vi "Four loops-one value from inner loop-HuYang.vi"(0 "File or Folder Path":path=path "P:/expt/PPMS data/SA03074H.20180120/14-rf1-rf2-9T", 5 "offset for each\n SG1 loop":i32, 7 "length X":i32=126, 9 "index":T1={"A"=10, "B"=1, "C"=2, "D"=0, "E"=10, "N1"=0, "N2"=0, "N3"=0, "N4"=0}, 11 "stop":bool, 12 "file contains 2D data?":bool) -> (4 "A vs B":cluster{i32[], dbl[]}[](graph), 6 "C vs D":cluster{dbl[], dbl[]}[](graph), 8 "E":dbl[][](graph), 10 "N":cluster{"N1":dbl, "N2":dbl, "N3":dbl, "N4":dbl}={"N1"=3599514757.669291, "N2"=3599514757.669291, "N3"=3599514757.669291, "N4"=3599514757.669291} {"N4" format="%#_6p"; "N3" format="%#_6p"; "N2" format="%#_6p"; "N1" format="%#_6p"}, 14 "Comments":string="IGOR\nX// Date: 1/22/2018 8:13 PM\nX// //Changed Voltage Femto from 20 dB to 80 dB (lock in channel 2)\nX// \nX// Stability diagram sweep\nX// \nX// Bias sweep: 0mV to 5mV, 2.5mV\nX// RF level sweep: - 4dBm, 2dBm\nX// DC2: -100 mV to 150mV, 2mV step\nX// DC1: -100 mV to 250mV, 1mV step\nX// \nX// B = 9T\nX// T = 50 mK\nX// Backgate = -0.1V \nX// \nX// I+: 5   0Vac + dc sweep, 13Hz, Sine wave\nX// I-: 28\nX// \nX// V1+/-: 4/27\nX// V2+/-: NA\nX// V3+/V3-: NA\nX// Vsg: 2&3\nX// \nX// 60 Hz prefilter off\nX// TC: 50m\nX// order:2\nX// SR830m sensitivity: 500uV\nX// \nX// I input gain: 1E+6\nX// V input gain:  10000appliedVsg= 0.000000\nX// appliedT= -4.000000appliedVsg= 0.150000\n\n\n\n\n\n\n\n\n\n\n\n\n\n\n\n\n\n\n\n\n\n\n\n\n\n\n\n\n\n\n\n\n\n\n\n\n\n\n\n\n\n\n\n\n\n\n\n\n\n\n\n\n\n\n\n\n\n\n\n\n\n\nX \nX Display/R 'time.SA03074H.000125'\nX AppendToGraph 'Vsg.SA03074H.000125'\nX AppendToGraph 'T.SA03074H.000125'\nX AppendToGraph 'B.SA03074H.000125'\nX AppendToGraph 'X0.SA03074H.000125'\nX AppendToGraph 'Y0.SA03074H.000125'\nX AppendToGraph 'X1.SA03074H.000125'\nX AppendToGraph 'Y1.SA03074H.000125'\nX AppendToGraph 'X2.SA03074H.000125'\nX AppendToGraph 'Y2.SA03074H.000125'\nX AppendToGraph 'X3.SA03074H.000125'\nX AppendToGraph 'Y3.SA03074H.000125'\nX AppendToGraph 'X4.SA03074H.000125'\nX AppendToGraph 'Y4.SA03074H.000125'\nX AppendToGraph 'X5.SA03074H.000125'\nX AppendToGraph 'Y5.SA03074H.000125'\nX AppendToGraph 'X6.SA03074H.000125'\nX AppendToGraph 'Y6.SA03074H.000125'\nX AppendToGraph 'X7.SA03074H.000125'\nX AppendToGraph 'Y7.SA03074H.000125'\nX AppendToGraph 'X8.SA03074H.000125'\nX AppendToGraph 'Y8.SA03074H.000125'\nX AppendToGraph 'X9.SA03074H.000125'\nX AppendToGraph 'Y9.SA03074H.000125'\nX AppendToGraph 'Gcalc.SA03074H.000125'\nX AppendToGraph '25.SA03074H.000125'\nX AppendToGraph '26.SA03074H.000125'\nX AppendToGraph '27.SA03074H.000125'\nX AppendToGraph '28.SA03074H.000125'\nX AppendToGraph '29.SA03074H.000125'\nX Label bottom \"x label\"\nX Label left \"y label\"\nX ModifyGraph rgb('time.SA03074H.000125')=(65280,0,0)\nX ModifyGraph rgb('Vsg.SA03074H.000125')=(65280,12288,0)\nX ModifyGraph rgb('T.SA03074H.000125')=(65280,23040,0)\nX ModifyGraph rgb('B.SA03074H.000125')=(65280,35328,0)\nX ModifyGraph rgb('X0.SA03074H.000125')=(65280,47616,0)\nX ModifyGraph rgb('Y0.SA03074H.000125')=(65280,58368,0)\nX ModifyGraph rgb('X1.SA03074H.000125')=(60416,65280,0)\nX ModifyGraph rgb('Y1.SA03074H.000125')=(48128,65280,0)\nX ModifyGraph rgb('X2.SA03074H.000125')=(37376,65280,0)\nX ModifyGraph rgb('Y2.SA03074H.000125')=(25088,65280,0)\nX ModifyGraph rgb('X3.SA03074H.000125')=(12800,65280,0)\nX ModifyGraph rgb('Y3.SA03074H.000125')=(2048,65280,0)\nX ModifyGraph rgb('X4.SA03074H.000125')=(0,65280,10240)\nX ModifyGraph rgb('Y4.SA03074H.000125')=(0,65280,22528)\nX ModifyGraph rgb('X5.SA03074H.000125')=(0,65280,33280)\nX ModifyGraph rgb('Y5.SA03074H.000125')=(0,65280,45568)\nX ModifyGraph rgb('X6.SA03074H.000125')=(0,65280,57856)\nX ModifyGraph rgb('Y6.SA03074H.000125')=(0,62464,65280)\nX ModifyGraph rgb('X7.SA03074H.000125')=(0,50176,65280)\nX ModifyGraph rgb('Y7.SA03074H.000125')=(0,37888,65280)\nX ModifyGraph rgb('X8.SA03074H.000125')=(0,27136,65280)\nX ModifyGraph rgb('Y8.SA03074H.000125')=(0,14848,65280)\nX ModifyGraph rgb('X9.SA03074H.000125')=(0,2560,65280)\nX ModifyGraph rgb('Y9.SA03074H.000125')=(8192,0,65280)\nX ModifyGraph rgb('Gcalc.SA03074H.000125')=(20480,0,65280)\nX ModifyGraph rgb('25.SA03074H.000125')=(32768,0,65280)\nX ModifyGraph rgb('26.SA03074H.000125')=(43520,0,65280)\nX ModifyGraph rgb('27.SA03074H.000125')=(55808,0,65280)\nX ModifyGraph rgb('28.SA03074H.000125')=(65280,0,62976)\nX ModifyGraph rgb('29.SA03074H.000125')=(65280,0,52224)\nX Legend/C/N=text0/J \"\\\\s('time.SA03074H.000125') time\\r\\\\s('Vsg.SA03074H.000125') Vsg\\r\\\\s('T.SA03074H.000125') T\\r\\\\s('B.SA03074H.000125') B\\r\\\\s('X0.SA03074H.000125') X0\\r\\\\s('Y0.SA03074H.000125') Y0\\r\\\\s('X1.SA03074H.000125') X1\\r\\\\s('Y1.SA03074H.000125') Y1\\r\\\\s('X2.SA03074H.000125') X2\\r\\\\s('Y2.SA03074H.000125') Y2\\r\\\\s('X3.SA03074H.000125') X3\\r\\\\s('Y3.SA03074H.000125') Y3\\r\\\\s('X4.SA03074H.000125') X4\\r\\\\s('Y4.SA03074H.000125') Y4\\r\\\\s('X5.SA03074H.000125') X5\\r\\\\s('Y5.SA03074H.000125') Y5\\r\\\\s('X6.SA03074H.000125') X6\\r\\\\s('Y6.SA03074H.000125') Y6\\r\\\\s('X7.SA03074H.000125') X7\\r\\\\s('Y7.SA03074H.000125') Y7\\r\\\\s('X8.SA03074H.000125') X8\\r\\\\s('Y8.SA03074H.000125') Y8\\r\\\\s('X9.SA03074H.000125') X9\\r\\\\s('Y9.SA03074H.000125') Y9\\r\\\\s('Gcalc.SA03074H.000125') Gcalc\"\nX ModifyGraph mirror(bottom)=1\nX ModifyGraph width=216\nX ModifyGraph height={Aspect,0.6}\nX ModifyGraph Log(bottom)=0\nX ModifyGraph Log(left)=0\nX \n")   [LabVIEW 2016]
uses:
  <vilib>/Utility/miscctls.llb/LVOffsetAndMultiplierTypeDef.ctl
panel:
  in  "length Y":i32
  in  "Index of inner loop":i32
  in  "D  is time?":bool
  in  "B is time?":bool
  out "time":string[][](table)=[["1/22/2018", "5:40 PM"], ["1/22/2018", "5:41 PM"], ["1/22/2018", "5:42 PM"], ["1/22/2018", "5:43 PM"], ["1/22/2018", "5:44 PM"], ["1/22/2018", "5:46 PM"], ["1/22/2018", "5:47 PM"], ["1/22/2018", "5:48 PM"], ["1/22/2018", "5:49 PM"], ["1/22/2018", "5:51 PM"], ["1/22/2018", "5:52 PM"], ["1/22/2018", "5:53 PM"], ["1/22/2018", "5:54 PM"], ["1/22/2018", "5:55 PM"], ["1/22/2018", "5:57 PM"], ["1/22/2018", "5:58 PM"], ["1/22/2018", "5:59 PM"], ["1/22/2018", "6:00 PM"], ["1/22/2018", "6:02 PM"], ["1/22/2018", "6:03 PM"], ["1/22/2018", "6:04 PM"], ["1/22/2018", "6:05 PM"], ["1/22/2018", "6:07 PM"], ["1/22/2018", "6:08 PM"], ["1/22/2018", "6:09 PM"], ["1/22/2018", "6:10 PM"], ["1/22/2018", "6:11 PM"], ["1/22/2018", "6:13 PM"], ["1/22/2018", "6:14 PM"], ["1/22/2018", "6:15 PM"], ["1/22/2018", "6:16 PM"], ["1/22/2018", "6:18 PM"], ["1/22/2018", "6:19 PM"], ["1/22/2018", "6:20 PM"], ["1/22/2018", "6:21 PM"], ["1/22/2018", "6:23 PM"], ["1/22/2018", "6:24 PM"], ["1/22/2018", "6:25 PM"], ["1/22/2018", "6:26 PM"], ["1/22/2018", "6:27 PM"], ["1/22/2018", "6:29 PM"], ["1/22/2018", "6:30 PM"], ["1/22/2018", "6:31 PM"], ["1/22/2018", "6:32 PM"], ["1/22/2018", "6:34 PM"], ["1/22/2018", "6:35 PM"], ["1/22/2018", "6:36 PM"], ["1/22/2018", "6:37 PM"], ["1/22/2018", "6:39 PM"], ["1/22/2018", "6:40 PM"], ["1/22/2018", "6:41 PM"], ["1/22/2018", "6:42 PM"], ["1/22/2018", "6:43 PM"], ["1/22/2018", "6:45 PM"], ["1/22/2018", "6:46 PM"], ["1/22/2018", "6:47 PM"], ["1/22/2018", "6:48 PM"], ["1/22/2018", "6:50 PM"], ["1/22/2018", "6:51 PM"], ["1/22/2018", "6:52 PM"], ["1/22/2018", "6:53 PM"], ["1/22/2018", "6:55 PM"], ["1/22/2018", "6:56 PM"], ["1/22/2018", "6:57 PM"], ["1/22/2018", "6:58 PM"], ["1/22/2018", "6:59 PM"], ["1/22/2018", "7:01 PM"], ["1/22/2018", "7:02 PM"], ["1/22/2018", "7:03 PM"], ["1/22/2018", "7:04 PM"], ["1/22/2018", "7:06 PM"], ["1/22/2018", "7:07 PM"], ["1/22/2018", "7:08 PM"], ["1/22/2018", "7:09 PM"], ["1/22/2018", "7:11 PM"], ["1/22/2018", "7:12 PM"], ["1/22/2018", "7:13 PM"], ["1/22/2018", "7:14 PM"], ["1/22/2018", "7:15 PM"], ["1/22/2018", "7:17 PM"], ["1/22/2018", "7:18 PM"], ["1/22/2018", "7:19 PM"], ["1/22/2018", "7:20 PM"], ["1/22/2018", "7:22 PM"], ["1/22/2018", "7:23 PM"], ["1/22/2018", "7:24 PM"], ["1/22/2018", "7:25 PM"], ["1/22/2018", "7:27 PM"], ["1/22/2018", "7:28 PM"], ["1/22/2018", "7:29 PM"], ["1/22/2018", "7:30 PM"], ["1/22/2018", "7:32 PM"], ["1/22/2018", "7:33 PM"], ["1/22/2018", "7:34 PM"], ["1/22/2018", "7:35 PM"], ["1/22/2018", "7:36 PM"], ["1/22/2018", "7:38 PM"], ["1/22/2018", "7:39 PM"], ["1/22/2018", "7:40 PM"], ["1/22/2018", "7:41 PM"], ["1/22/2018", "7:43 PM"], ["1/22/2018", "7:44 PM"], ["1/22/2018", "7:45 PM"], ["1/22/2018", "7:46 PM"], ["1/22/2018", "7:48 PM"], ["1/22/2018", "7:49 PM"], ["1/22/2018", "7:50 PM"], ["1/22/2018", "7:51 PM"], ["1/22/2018", "7:52 PM"], ["1/22/2018", "7:54 PM"], ["1/22/2018", "7:55 PM"], ["1/22/2018", "7:56 PM"], ["1/22/2018", "7:57 PM"], ["1/22/2018", "7:59 PM"], ["1/22/2018", "8:00 PM"], ["1/22/2018", "8:01 PM"], ["1/22/2018", "8:02 PM"], ["1/22/2018", "8:04 PM"], ["1/22/2018", "8:05 PM"], ["1/22/2018", "8:06 PM"], ["1/22/2018", "8:07 PM"], ["1/22/2018", "8:08 PM"], ["1/22/2018", "8:10 PM"], ["1/22/2018", "8:11 PM"], ["1/22/2018", "8:12 PM"], ["1/22/2018", "8:13 PM"]]
  in  "Use Folder Index File?":bool
  in  "Generate Folder Index File?":bool
  in  "Ez name":string="Ix (nA)"
  in  "Ey name":string="DC2 (V)"
  in  "Ex name":string="DC1 (V)"
  in  "C y name":string="C y name"
  in  "D x name":string="D x name"
  in  "A y name":string="Ix (nA)"
  in  "B x name":string="DC1 (V)"
  out "Index, Wavenames":string[][](table)=[["0", "'time.SA03074H.000125'\n"], ["1", "'Vsg.SA03074H.000125'\n"], ["2", "'T.SA03074H.000125'\n"], ["3", "'B.SA03074H.000125'\n"], ["4", "'X0.SA03074H.000125'\n"], ["5", "'Y0.SA03074H.000125'\n"], ["6", "'X1.SA03074H.000125'\n"], ["7", "'Y1.SA03074H.000125'\n"], ["8", "'X2.SA03074H.000125'\n"], ["9", "'Y2.SA03074H.000125'\n"], ["10", "'X3.SA03074H.000125'\n"], ["11", "'Y3.SA03074H.000125'\n"], ["12", "'X4.SA03074H.000125'\n"], ["13", "'Y4.SA03074H.000125'\n"], ["14", "'X5.SA03074H.000125'\n"], ["15", "'Y5.SA03074H.000125'\n"], ["16", "'X6.SA03074H.000125'\n"], ["17", "'Y6.SA03074H.000125'\n"], ["18", "'X7.SA03074H.000125'\n"], ["19", "'Y7.SA03074H.000125'\n"], ["20", "'X8.SA03074H.000125'\n"], ["21", "'Y8.SA03074H.000125'\n"], ["22", "'X9.SA03074H.000125'\n"], ["23", "'Y9.SA03074H.000125'\n"], ["24", "'Gcalc.SA03074H.000125'\n"], ["25", "'25.SA03074H.000125'\n"], ["26", "'26.SA03074H.000125'\n"], ["27", "'27.SA03074H.000125'\n"], ["28", "'28.SA03074H.000125'\n"], ["29", "'29.SA03074H.000125'\n"], ["", ""]]
  in  "recolor traces?":bool
  in  "Ex":T2={"Offset"=-0.1, "Multiplier"=0.001}
  in  "Ey":T2={"Offset"=-0.1, "Multiplier"=0.002}
  out "Path":path=path "P:/expt/PPMS data/SA03074H.20180120/14-rf1-rf2-9T/SA03074H.000125.itx"
  out "counter":i32=125
  in  "pattern":string="*.itx"
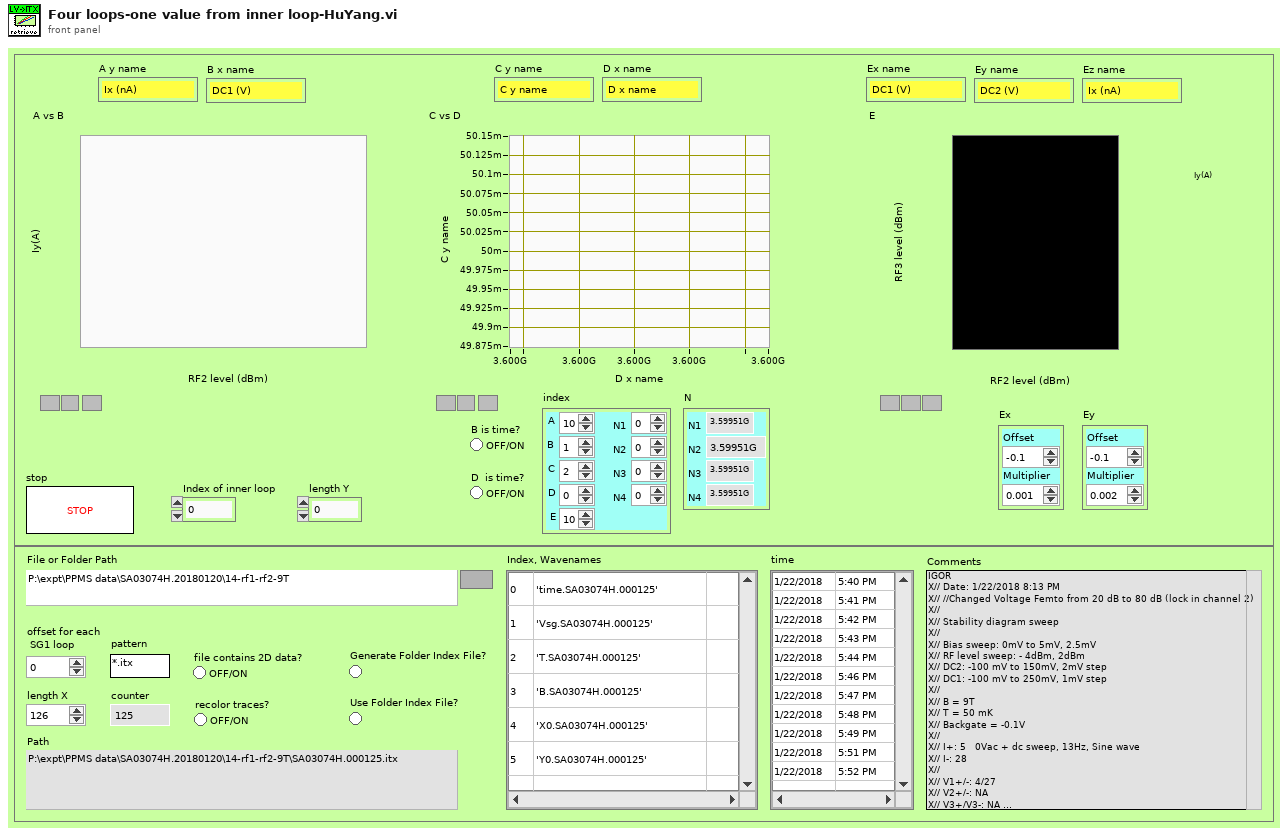
[diagram p1: front panel]
types:
  T1 = cluster{"A":i32, "B":i32, "C":i32, "D":i32, "E":i32, "N1":i32, "N2":i32, "N3":i32, "N4":i32}
  T2 = typedef "LVOffsetAndMultiplierTypeDef.ctl" = cluster{"Offset":dbl, "Multiplier":dbl}
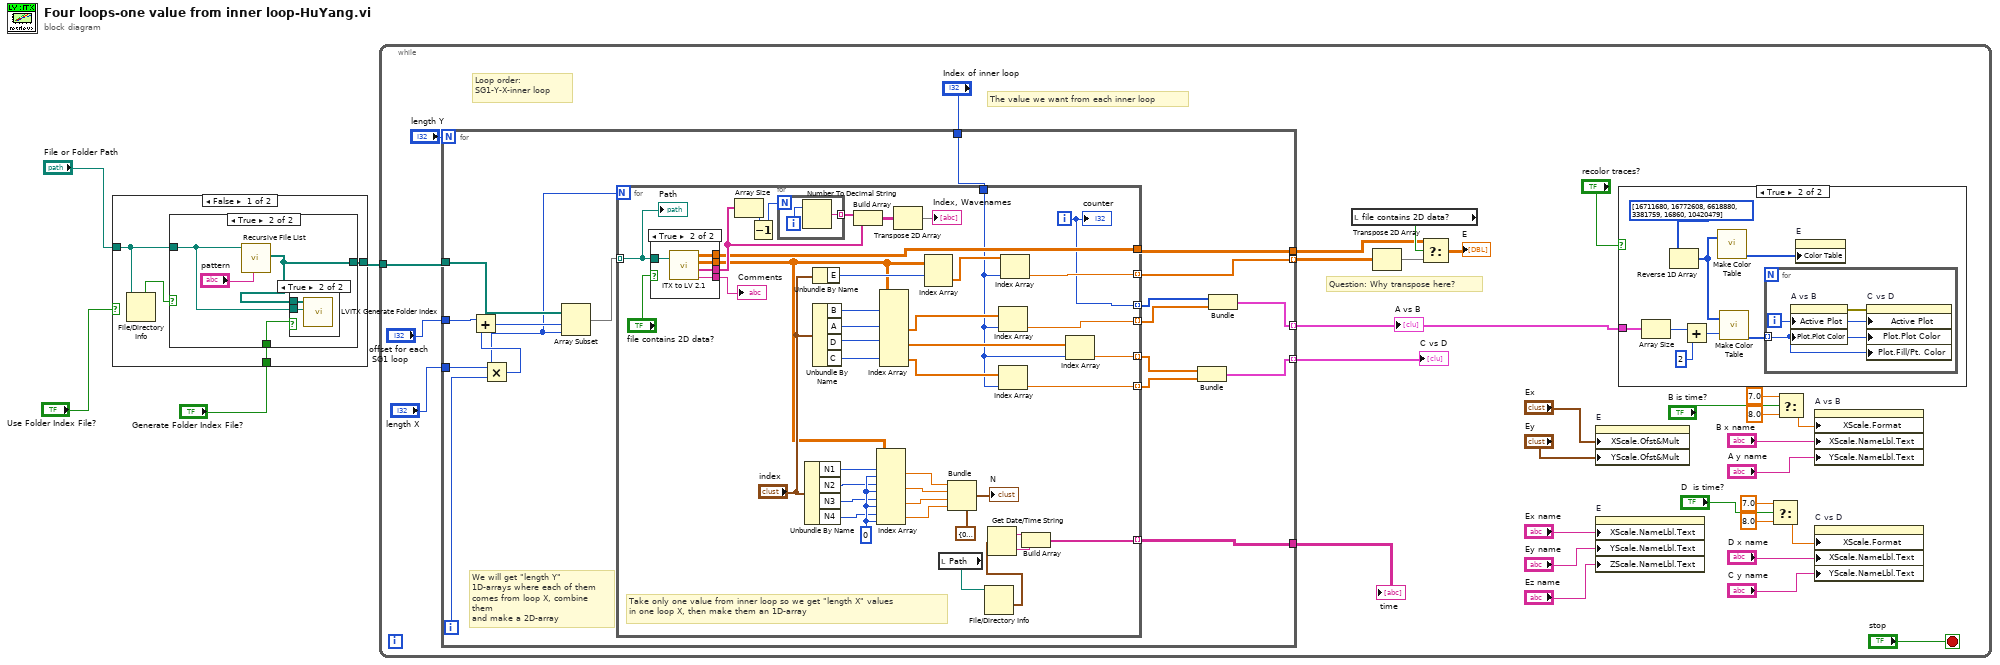
[diagram p0: block diagram]
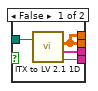
[diagram p2: hidden frame]
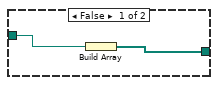
[diagram p4: hidden frame]
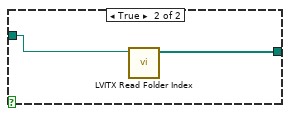
[diagram p6: hidden frame]
diagram:
  n1 = case shown="False" "Use Folder Index File?" {
    tunnel: [w6 w17] -> w2
    tunnel: "File or Folder Path" -> [w8 w18]
    tunnel: "Generate Folder Index File?" -> [w5 _]
    frame False {
      n2 = File/Directory Info(path=w8) -> (directory=w7:bool)  [unwired: 1 in, 6 out]
      n3 = case shown="True" w7 {
        tunnel: [w10 w13] -> w6
        tunnel: w8 -> [w9 w12]
        tunnel: w5 -> [_ w11]
        frame False {
          n4 = Build Array(w9) -> (w10:path[])
        }
        frame True {
          n5 = call <vilib>:"Recursive File List.vi"("pattern"="pattern", "Folder Path"=w12) -> ("All Files in Dir"=w13:path[])  [unwired: 5 in, 4 out]
          n6 = case shown="True" w11 {
            tunnel: w13 -> [_ w16]
            tunnel: w12 -> [_ w15]
            frame False {
            }
            frame True {
              n7 = call <userlib>:"LVITX Generate Folder Index.vi"("File or Folder Path"=w15, "All Files in Dir"=w16) -> ()  [unwired: 10 in]
            }
          }
        }
      }
    }
    frame True {
      n8 = call <userlib>:"LVITX Read Folder Index.vi"("File or Folder Path"=w18) -> ("Array"=w17:path[])  [unwired: 10 in]
    }
  }
  n9 = while {
    tunnel: w2 -> [w22]
    stop <- "stop" stop-if-true
    # "Question: Why transpose here?"
    # "The value we want from each inner loop"
    # "Loop order:\nSG1-Y-X-inner loop"
    n10 = for {
      N: "length Y" -> [_]
      tunnel: [w58] -> w46 mode=indexing
      tunnel: [w67] -> w44
      tunnel: [w57] -> w42 mode=indexing
      tunnel: [w56] -> w41 mode=indexing
      tunnel: [w66] -> w33
      tunnel: w22 -> [w64]
      tunnel: "Index of inner loop" -> [w65]
      tunnel: "offset for each\n SG1 loop" -> [w62]
      tunnel: "length X" -> [w59]
      i -> [w53]
      # "We will get \"length Y\" 1D-arrays where each of them comes from loop X, combine them \nand make a 2D-array"
      n11 = Multiply(x=w59, y=w53) -> (x*y=w63:i32)
      n12 = Add(x=w62, y=w63) -> (x+y=w61:i32)
      n13 = Array Subset(array=w64, index=w61, length=w59) -> (w60:path[])
      n14 = for {
        N: w59 -> [_]
        tunnel: w60 -> [w109] mode=indexing
        tunnel: [w109] -> _ mode=indexing
        tunnel: [w101] -> w67
        tunnel: [w78] -> w66 mode=indexing
        tunnel: w65 -> [w72]
        tunnel: [w76] -> w58 mode=indexing
        tunnel: [w68] -> w52 mode=indexing
        tunnel: [w69] -> w51 mode=indexing
        tunnel: [w71] -> w54 mode=indexing
        tunnel: [w70] -> w55 mode=indexing
        i -> [w68]
        w100 = 0 ("disabled index (col)")
        # "Take only one value from inner loop so we get \"length X\" values \nin one loop X, then make them an 1D-array"
        n15 = case shown="True" "file contains 2D data?" {
          tunnel: [w116 w119] -> w110
          tunnel: [w114 w120] -> w82
          tunnel: w109 -> [w115 w121]
          tunnel: [w113 w118] -> w102
          tunnel: [w114 w117] -> w101
          frame False {
            n16 = call <userlib>:"ITX to LV 2.1 1D.vi"("file (use dialog)"=w115) -> ("1D arrays"=w114:dbl[][], "wave names"=w113:string[], "Notes"=w116:string)  [unwired: 2 in]
          }
          frame True {
            n17 = call <userlib>:"ITX to LV 2.1.vi"("file (use dialog)"=w121) -> ("2D array"=w117:dbl[][], "1D arrays"=w120:dbl[][], "wave names"=w118:string[], "Notes"=w119:string)  [unwired: 1 in]
          }
        }
        "Comments" <- w110
        n18 = Array Size(array=w102) -> (size(s)=w105:i32)
        n19 = Decrement(x=w105) -> (x-1=w104:i32)
        n20 = for {
          N: w104 -> [_]
          tunnel: [w111] -> w107 mode=indexing
          i -> [w112]
          n21 = Number To Decimal String(number=w112) -> (decimal integer string=w111:string)  [unwired: 1 in]
        }
        n22 = Unbundle By Name("index") -> ("N1"=w93:i32, "N2"=w94:i32, "N3"=w95:i32, "N4"=w96:i32)
        n23 = Unbundle By Name("index") -> ("E"=w92:i32)
        n24 = Unbundle By Name("index") -> ("B"=w91:i32, "A"=w90:i32, "D"=w89:i32, "C"=w88:i32)
        n25 = Build Array(w107, w102) -> (w103:string[][])
        n26 = Index Array(array=w82, index (row) #1=w93, index (col) #1=w100, index (row) #2=w94, index (col) #2=w100, index (row) #3=w95, index (col) #3=w100, index (row) #4=w96, index (col) #4=w100) -> (element #1=w83:dbl, element #2=w84:dbl, element #3=w85:dbl, element #4=w99:dbl)
        n27 = Index Array(array=w82, index (row) #1=w91, index (row) #2=w90, index (row) #3=w89, index (row) #4=w88) -> (element #2=w75:dbl[], element #3=w74:dbl[], element #4=w73:dbl[])  [unwired: 4 in, 1 out]
        n28 = Transpose 2D Array(2D array=w103) -> (transposed array=→"Index, Wavenames":string[][])
        n29 = Index Array(array=w82, index (row)=w92) -> (element=w77:dbl[])  [unwired: 1 in]
        n30 = local read "Path"() -> (w86:path)
        n31 = Bundle(cluster=cluster{"N1":dbl, "N2":dbl, "N3":dbl, "N4":dbl} {"N1"=0.0, "N2"=0.0, "N3"=0.0, "N4"=0.0}, "N1"=w83, "N2"=w84, "N3"=w85, "N4"=w99) -> (→"N":cluster{"N1":dbl, "N2":dbl, "N3":dbl, "N4":dbl})
        n32 = File/Directory Info(path=w86) -> (last mod=w81:timestamp)  [unwired: 1 in, 6 out]
        n33 = Get Date/Time String(seconds (now)=w81) -> (date string=w80:string, time string=w79:string)  [unwired: 2 in]
        n34 = Index Array(array=w75, index=w72) -> (element=w69:dbl)
        n35 = Index Array(array=w73, index=w72) -> (element=w71:dbl)
        n36 = Index Array(array=w77, index=w72) -> (element=w76:dbl)
        n37 = Build Array(w80, w79) -> (w78:string[])
        n38 = Index Array(array=w74, index=w72) -> (element=w70:dbl)
        "counter" <- w68
        "Path" <- w109
      }
      n39 = Bundle(w55, w54) -> (w56:cluster{dbl[], dbl[]})  [unwired: 1 in]
      n40 = Bundle(w52, w51) -> (w57:cluster{i32[], dbl[]})  [unwired: 1 in]
    }
    "A vs B" <- w42
    "C vs D" <- w41
    "time" <- w33
    n41 = local read "file contains 2D data?"() -> (w49:bool)
    n42 = Transpose 2D Array(2D array=w46) -> (transposed array=w47:dbl[][])
    n43 = Select(t=w44, s=w49, f=w47) -> (s? t:f=→"E":dbl[][])
    n44 = property on="E" class="IntGraph (strict)"("XScale.Ofst&Mult"="Ex", "YScale.Ofst&Mult"="Ey") -> ()  [unwired: 2 in, 2 out]
    n45 = property on="E" class="IntGraph (strict)"("XScale.NameLbl.Text"="Ex name", "YScale.NameLbl.Text"="Ey name", "ZScale.NameLbl.Text"="Ez name") -> ()  [unwired: 2 in, 2 out]
    n46 = case shown="True" "recolor traces?" {
      tunnel: w42 -> [_ w124]
      frame False {
      }
      frame True {
        n47 = Array Size(array=w124) -> (size(s)=w125:i32)
        n48 = Reverse 1D Array(array=u32[] [16711680, 16772608, 6618880, 3381759, 16860, 10420479] ("color scale")) -> (reversed array=w123:u32[])
        n49 = Add(x=w125, y=2 ("x")) -> (x+y=w129:i32)
        n50 = call <userlib>:"Make Color Table.vi"("Array"=w123) -> ("Color Tbl"=w127:u32[])  [unwired: 1 in, 3 out]
        n51 = call <userlib>:"Make Color Table.vi"("Array"=w123, "Size/3"=w129) -> ("Color Tbl"=w126:u32[])  [unwired: 3 out]
        n52 = for {
          tunnel: w126 -> [w130] mode=indexing
          i -> [w131]
          n53 = property on="A vs B" class="XYGraph (strict)"("Active Plot"=w131, "Plot.Plot Color"=w130) -> (error out=w132:errorcluster)  [unwired: 2 in, 1 out]
          n54 = property on="C vs D" class="XYGraph (strict)"(error in=w132, "Active Plot"=w131, "Plot.Plot Color"=w130, "Plot.Fill/Pt. Color"=w130) -> ()  [unwired: 1 in, 2 out]
        }
        n55 = property on="E" class="IntGraph (strict)"("Color Table"=w127) -> ()  [unwired: 2 in, 2 out]
      }
    }
    n56 = Select(t=7.0, s="D  is time?", f=8.0) -> (s? t:f=w29:dbl)
    n57 = Select(t=7.0, s="B is time?", f=8.0) -> (s? t:f=w30:dbl)
    n58 = property on="A vs B" class="XYGraph (strict)"("XScale.Format"=w30, "XScale.NameLbl.Text"="B x name", "YScale.NameLbl.Text"="A y name") -> ()  [unwired: 2 in, 2 out]
    n59 = property on="C vs D" class="XYGraph (strict)"("XScale.Format"=w29, "XScale.NameLbl.Text"="D x name", "YScale.NameLbl.Text"="C y name") -> ()  [unwired: 2 in, 2 out]
  }
